vi "DSF.Engine.Memory.Cache.Transfer Group.Create.vi"(7 "Transfer Cache type":refnum<class "DSF.Engine.Memory.Cache.Transfer.lvclass">, 8 "error in (no error)":errorcluster, 10 "Transfer Group Configuration":refnum<class "DSF.Shared.Configuration.Transfer Group.lvclass">, 11 "Transfer Group Cache type":refnum<class "DSF.Engine.Memory.Cache.Transfer Group.lvclass">) -> (0 "error out":errorcluster, 3 "Transfer Group Cache":refnum<class "DSF.Engine.Memory.Cache.Transfer Group.lvclass">)   [LabVIEW 2016, in "DSF.Engine.lvlib" / "DSF.Engine.Memory.Cache.Transfer Group.lvclass"]
uses:
  DSF.Engine.Memory.Cache.Transfer Group.lvclass
  DSF.Engine.Memory.Cache.Transfer.lvclass
  Shared/Classes/Transfer Group/DSF.Shared.Configuration.Transfer Group.lvclass
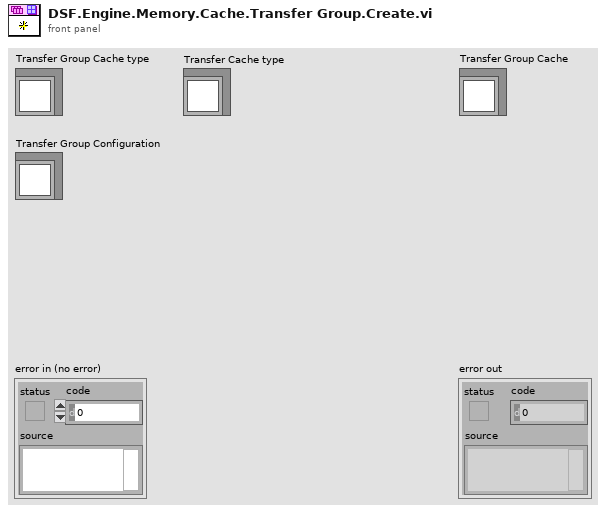
[diagram p1: front panel]
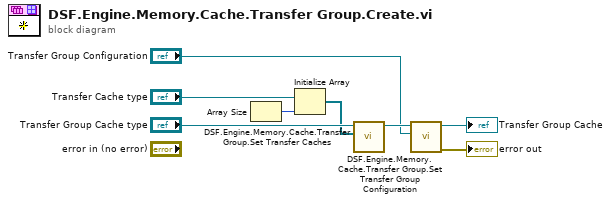
[diagram p0: block diagram]
diagram:
  n1 = Array Size() -> (size(s)=w8:i32)  [unwired: 1 in]
  n2 = Initialize Array("Transfer Cache type", w8) -> (w5:refnum<class "DSF.Engine.Memory.Cache.Transfer.lvclass">[])
  n3 = call "DSF.Engine.Memory.Cache.Transfer Group.Set Transfer Caches.vi"("Transfer Caches"=w5, "Transfer Group Cache in"="Transfer Group Cache type") -> ("Transfer Group Cache out"=w4:refnum<class "DSF.Engine.Memory.Cache.Transfer Group.lvclass">)  [unwired: 9 in]
  n4 = call "DSF.Engine.Memory.Cache.Transfer Group.Set Transfer Group Configuration.vi"("Transfer Group Configuration"="Transfer Group Configuration", "Transfer Group Cache in"=w4) -> ("error out"=→"error out":errorcluster, "Transfer Group Cache out"=→"Transfer Group Cache":refnum<class "DSF.Engine.Memory.Cache.Transfer Group.lvclass">)  [unwired: 8 in]
